vi "INTOCODE.vi"(7 "CODE_MAIN":string, 9 "PRODUCT_ID":string, 11 "错误输入":errorcluster) -> (15 "error out":errorcluster)   [LabVIEW 2020]
panel:
  in  "USER_ID":string
  in  "DEVICE_ID":string
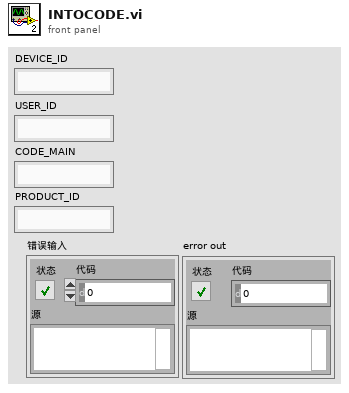
[diagram p1: front panel]
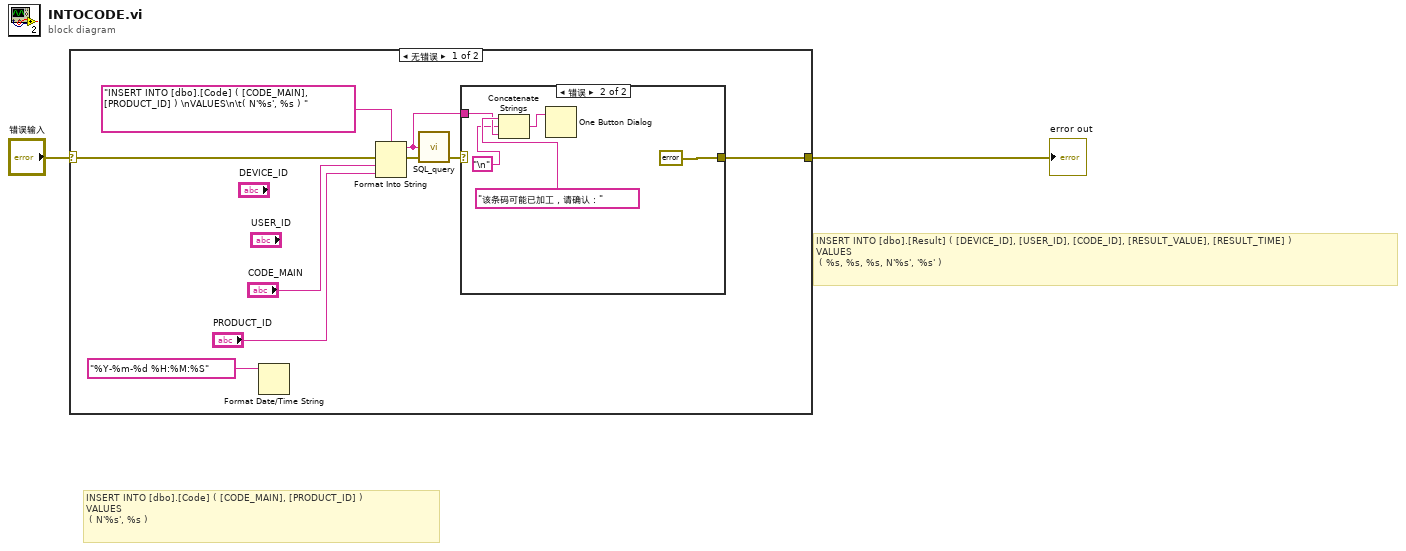
[diagram p0: block diagram]
diagram:
  # "INSERT INTO [dbo].[Code] ( [CODE_MAIN], [PRODUCT_ID] ) \nVALUES\n\t( N'%s', %s )"
  # "INSERT INTO [dbo].[Result] ( [DEVICE_ID], [USER_ID], [CODE_ID], [RESULT_VALUE], [RESULT_TIME] ) \nVALUES\n\t( %s, %s, %s, N'%s', '%s' )"
  n1 = case shown="无错误" "错误输入" {
    selector: "错误输入" -> [w6 w18]
    tunnel: [w3 w18] -> w1
    frame No Error {
      n2 = Format Date/Time String(time format string (%c)="%Y-%m-%d %H:%M:%S" ("时间格式字符串(%c)")) -> ()  [unwired: 2 in, 1 out]
      n3 = Format Into String(format string="INSERT INTO [dbo].[Code] ( [CODE_MAIN], [PRODUCT_ID] ) \nVALUES\n\t( N'%s', %s ) ", error in=w6, "CODE_MAIN", "PRODUCT_ID") -> (resulting string=w4:string, error out=w11:errorcluster)  [unwired: 1 in]
      n4 = call "SQL_query.vi"("error in (no error)"=w11, "SQL query"=w4) -> ("error out"=w5:errorcluster)  [unwired: 2 in, 1 out]
      n5 = case shown="错误" w5 {
        selector: w5 -> [w12 _]
        tunnel: w4 -> [_ w14]
        tunnel: [w12 errorcluster {"status"=FALSE, "code"=0, "source"=""} ("error IO")] -> w3
        frame No Error {
        }
        frame Error {
          n6 = Concatenate Strings("该条码可能已加工，请确认：", "\n", w14) -> (w16:string)
          n7 = One Button Dialog(message=w16) -> ()  [unwired: 1 in, 1 out]
        }
      }
    }
    frame Error {
    }
  }
  "error out" <- w1
